vi "Create Native_SuBUS Waveform.vi"(7 "sample rate":dbl=20000000.0 format="%#_6p", 8 "error in (no error)":errorcluster, 9 "Reg_Address_Data":T2={"Address"=81, "Data"=0} {"Address" format="%.0x"}, 10 "USID":T1=13 max=15 format="%.0x", 11 "OVS":u8=16) -> (0 "error out":errorcluster, 3 "Digital Waveform Graph":digitalwaveform(graph))   [LabVIEW 2013]
uses:
  XP2100/Controls/Reg_Address_Data.ctl
  XP2100/Controls/USID.ctl
  <vilib>/Waveform/DWDTOps.llb/DWDT Append Digital Samples.vi
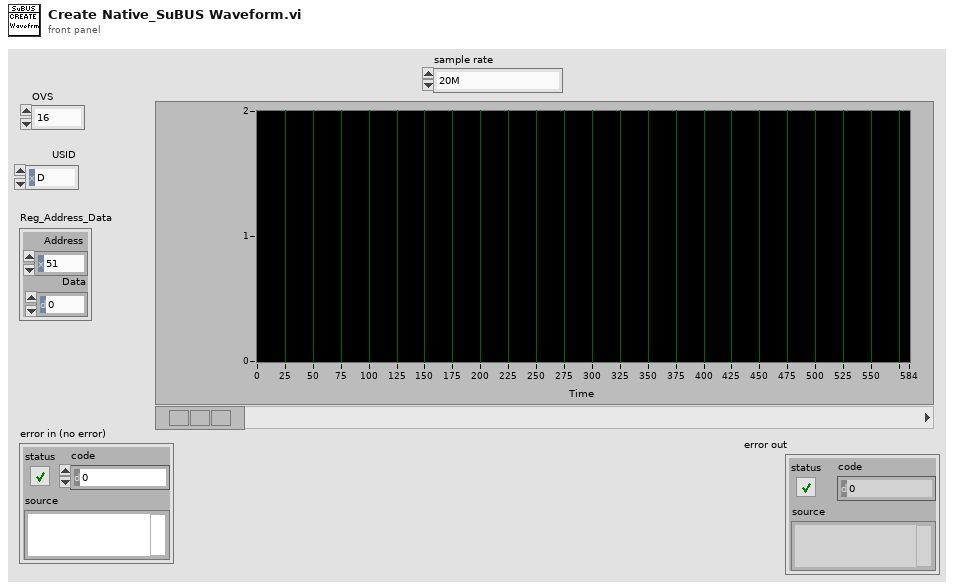
[diagram p1: front panel]
types:
  T1 = typedef "USID.ctl" = u8
  T2 = typedef "Reg_Address_Data.ctl" = cluster{"Address":u8, "Data":u8}
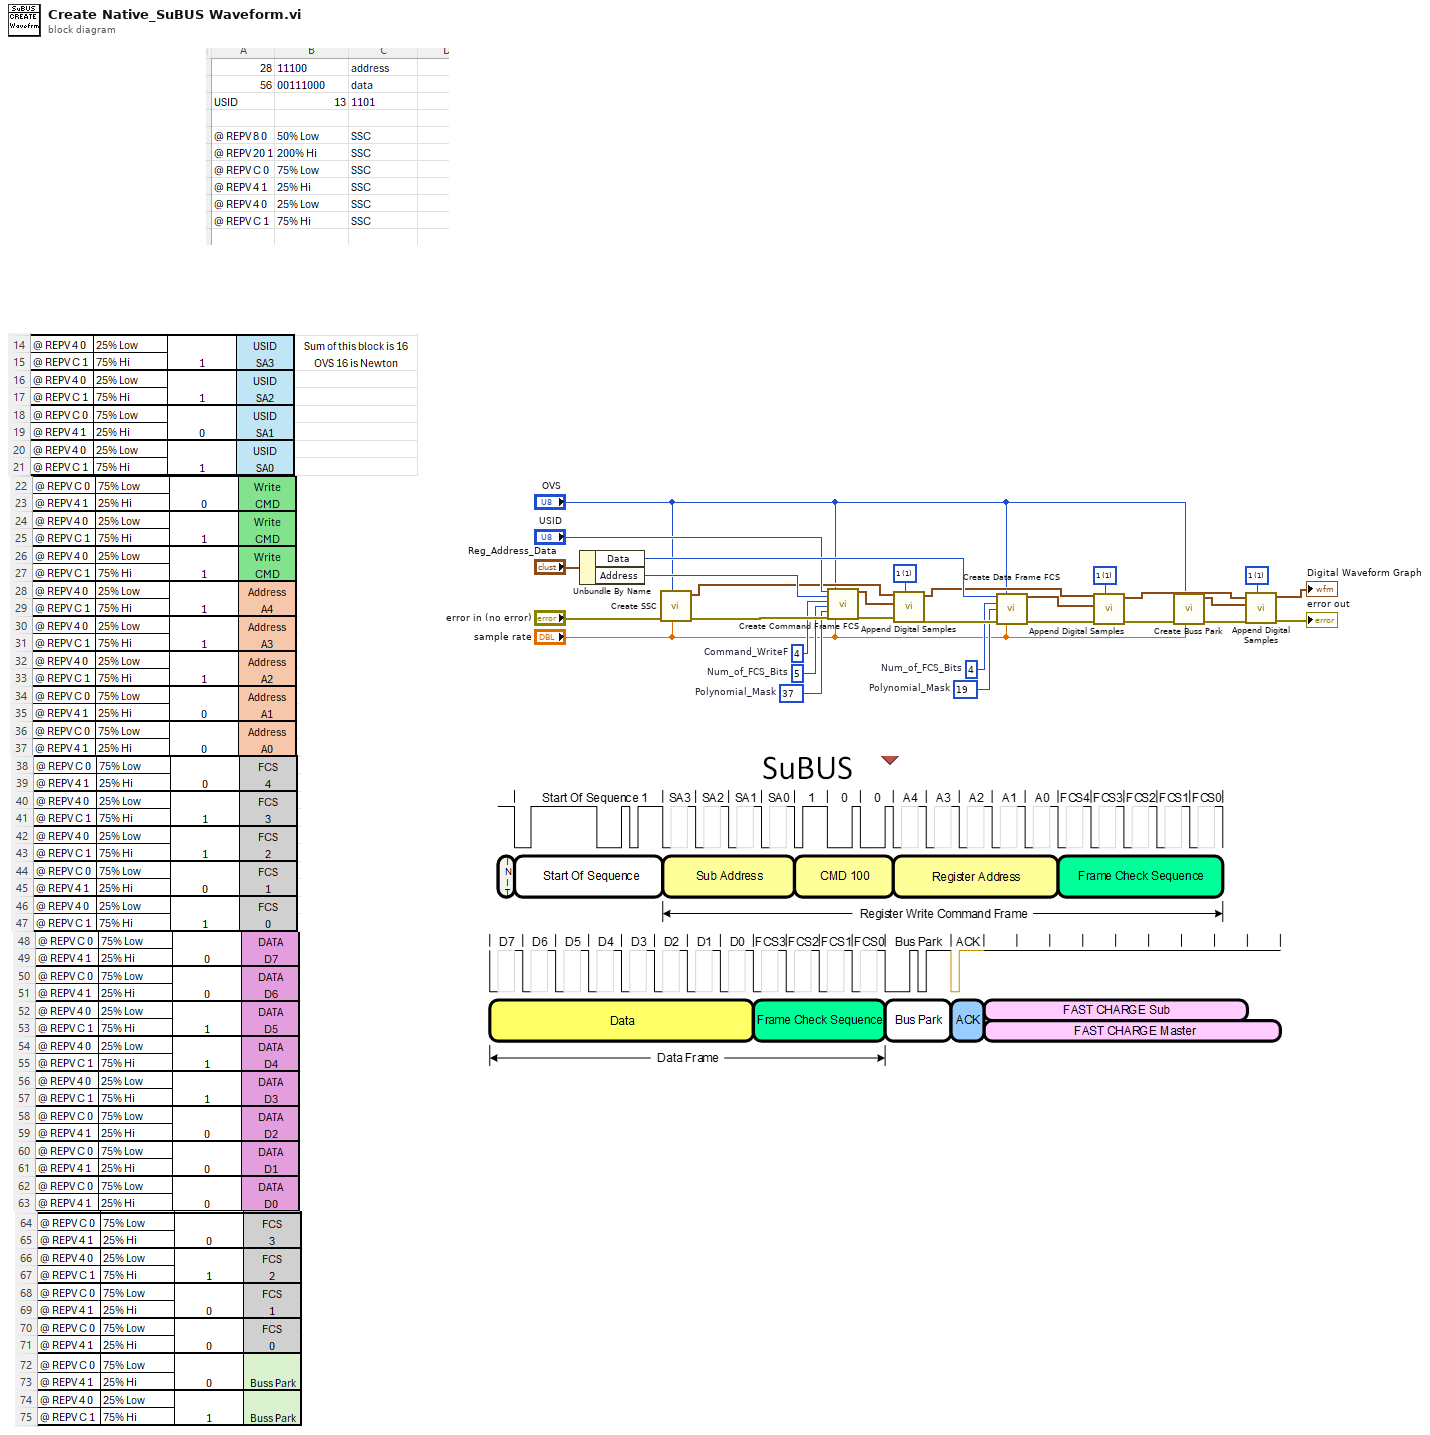
[diagram p0: block diagram]
diagram:
  w8 = u8 1 items=["0", "1", "Z", "L", "H", "X", "T", "V"] ("default value")
  w24 = u8 19  # Polynomial_Mask
  w23 = u8 4  # Num_of_FCS_Bits
  w26 = u8 1 items=["0", "1", "Z", "L", "H", "X", "T", "V"] ("default value")
  w28 = u8 1 items=["0", "1", "Z", "L", "H", "X", "T", "V"] ("default value")
  w19 = u8 37  # Polynomial_Mask
  w17 = u8 4  # Command_WriteF
  w18 = u8 5  # Num_of_FCS_Bits
  n1 = Unbundle By Name("Reg_Address_Data") -> ("Data"=w22:u8, "Address"=w15:u8)
  n2 = call "Create SSC.vi"("sample rate"="sample rate", "OVS"="OVS", "error in (no error)"="error in (no error)") -> ("error out"=w20:errorcluster, "Digital Waveform Graph"=w5:digitalwaveform)  [unwired: 7 in]
  n3 = call "Create Command Frame FCS.vi"("USID"="USID", "Address"=w15, "Command_WriteF"=w17, "Num_of_FCS_Bits"=w18, "Polynomial_Mask"=w19, "error in (no error)"=w20, "OVS"="OVS", "sample rate"="sample rate") -> ("Digital Waveform Graph_Out"=w7:digitalwaveform, "error out"=w14:errorcluster)  [unwired: 10 in]
  n4 = call-poly <vilib>:"Append Digital Samples.vi"("default value"=w28, "error in (no error)"=w14, "digital waveform B"=w7, "digital waveform A"=w5) -> ("error out"=w27:errorcluster, "digital waveform out"=w6:digitalwaveform)  [unwired: 6 in]
  n5 = call "Create Data Frame FCS.vi"("Data"=w22, "OVS"="OVS", "Num_of_FCS_Bits"=w23, "Polynomial_Mask"=w24, "error in (no error)"=w27, "sample rate"="sample rate") -> ("Digital Waveform Graph_Out"=w21:digitalwaveform, "error out"=w25:errorcluster)  [unwired: 8 in]
  n6 = call-poly <vilib>:"Append Digital Samples.vi"("default value"=w26, "error in (no error)"=w25, "digital waveform B"=w21, "digital waveform A"=w6) -> ("error out"=w12:errorcluster, "digital waveform out"=w10:digitalwaveform)  [unwired: 6 in]
  n7 = call "Create Buss Park.vi"("sample rate"="sample rate", "OVS"="OVS", "error in (no error)"=w12) -> ("error out"=w11:errorcluster, "Digital Waveform Graph"=w9:digitalwaveform)  [unwired: 7 in]
  n8 = call-poly <vilib>:"Append Digital Samples.vi"("default value"=w8, "error in (no error)"=w11, "digital waveform B"=w9, "digital waveform A"=w10) -> ("error out"=→"error out":errorcluster, "digital waveform out"=→"Digital Waveform Graph":digitalwaveform)  [unwired: 6 in]
